vi "DrawRobot.vi"(1 "(xr,yr) old":cluster{"x robot":dbl, "y robot":dbl}, 2 "(xr,yr) new":cluster{"x robot":dbl, "y robot":dbl}, 3 "2D Picture":picture) -> (0 "new picture":picture)   [LabVIEW 2010]
doc: "Draws a magenta circle at the curretn (x,y) coordinates of the Robot in the current mission definition file.\nInputs:\nPicture to draw on\nCluster X\n y coordinates of robot\nOutput:\nmodified picture"
panel:
  # "Draws a circle at the current x,y coordinates of the robot"
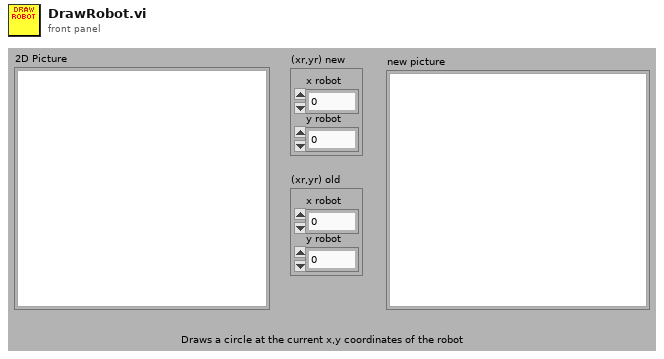
[diagram p1: front panel]
types:
  T1 = cluster{"Width":u16, "Style":enum32{"Solid", "Dash", "Dot", "DashDot", "DashDotDot"}}
  T2 = typedef "imagedata.ctl" = cluster{"image type":i32, "image depth":i32, "image":u8[], "mask":u8[], "colors":u32[], "Rectangle":cluster{"left":i16, "top":i16, "right":i16, "bottom":i16}}
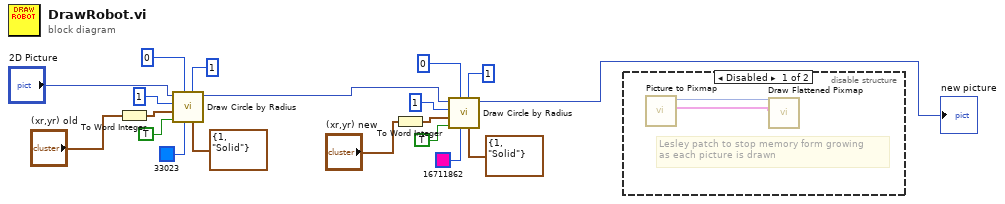
[diagram p0: block diagram]
diagram:
  n1 = To Word Integer(number="(xr,yr) old") -> (16bit integer=w5:cluster{"x robot":i16, "y robot":i16})
  n2 = call <vilib>:"Draw Circle by Radius.vi"("pen"=T1 {"Width"=1, "Style"=enum."Solid"}, "arc size(360)"=i16 1, "color(black)"=u32 33023, "start angle(0)"=i16 0, "fill?(F)"=TRUE, "pixel center"=w5, "radius"=i16 1, "picture"="2D Picture") -> ("new picture"=w1:picture)  [unwired: 3 in]
  n3 = To Word Integer(number="(xr,yr) new") -> (16bit integer=w19:cluster{"x robot":i16, "y robot":i16})
  n4 = call <vilib>:"Draw Circle by Radius.vi"("pen"=T1 {"Width"=1, "Style"=enum."Solid"}, "arc size(360)"=i16 1, "color(black)"=u32 16711862, "start angle(0)"=i16 0, "fill?(F)"=TRUE, "pixel center"=w19, "radius"=i16 1, "picture"=w1) -> ("new picture"=→"new picture":picture)  [unwired: 3 in]
  n5 = disable-structure shown="Disabled" {
    frame Disabled {
      # "Lesley patch to stop memory form growing\nas each picture is drawn"
      n6 = call <vilib>:"Picture to Pixmap.vi"() -> ("image data"=w20:T2, "new picture"=w21:picture)  [unwired: 10 in]
      n7 = call <vilib>:"Draw Flattened Pixmap.vi"("image data"=w20, "picture"=w21) -> ()  [unwired: 7 in, 1 out]
    }
    frame Enabled {
    }
  }
